vi "Robot Systems.vi"(11 "Robot Controls":T1) -> ()   [LabVIEW 2014]
uses:
  Robot Commands.ctl
panel:
  # "Field Centric"
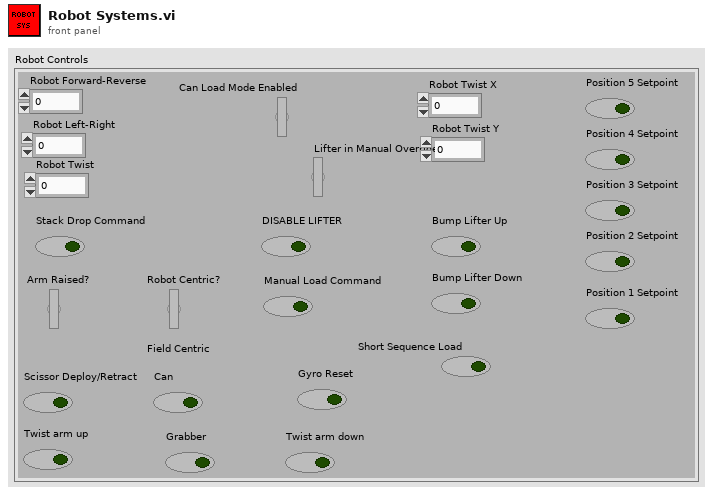
[diagram p1: front panel]
types:
  T1 = typedef "Robot Commands.ctl" = cluster{"Robot Forward-Reverse":dbl, "Robot Left-Right":dbl, "Robot Twist":dbl, "Can Load Mode Enabled":bool, "Lifter in Manual Override?":bool, "Stack Drop Command":bool, "Arm Raised?":bool, "DISABLE LIFTER":bool, "Position 1 Setpoint":bool, "Position 2 Setpoint":bool, "Position 3 Setpoint":bool, "Position 4 Setpoint":bool, "Position 5 Setpoint":bool, "Bump Lifter Down":bool, "Bump Lifter Up":bool, "Manual Load Command":bool, "Robot Centric?":bool, "Scissor Deploy/Retract":bool, "Grabber":bool, "Can":bool, "Twist arm up":bool, "Gyro Reset":bool, "Twist arm down":bool, "Short Sequence Load":bool, "Robot Twist X":dbl, "Robot Twist Y":dbl}
  T2 = typedef "Step Deployment SS State.ctl" = enum16{"Manual Override", "Disabled"}
  T3 = typedef "Stacking SS State.ctl" = enum16{"Manual Load", "Manual Override"}
  T4 = typedef "Drive SS State.ctl" = enum16{"Swerve Drive", "Arcade Drive", "Mecanum Drive"}
  T5 = typedef "Stacking SS Actuators.ctl" = cluster{"Can Solenoid":T6, "Lifter Motor":dbl, "Grabber Solenoid":T6}
  T6 = typedef "WPI_SolenoidValue.ctl" = enum16{"Off", "On", "Forward", "Reverse"}
  T7 = typedef "Drive SS Actuator Values.ctl" = cluster{"Front Left Drive Motor":dbl, "Front Left Spin Motor":dbl, "Front Right Drive Motor":dbl, "Front Right Spin Motor":dbl, "Rear Left Drive Motor":dbl, "Rear Left Spin Motor":dbl, "Rear Right Drive Motor":dbl, "Rear Right Spin Motor":dbl}
  T8 = typedef "Step Deployment Actuator Values.ctl" = cluster{"Scissors":T6}
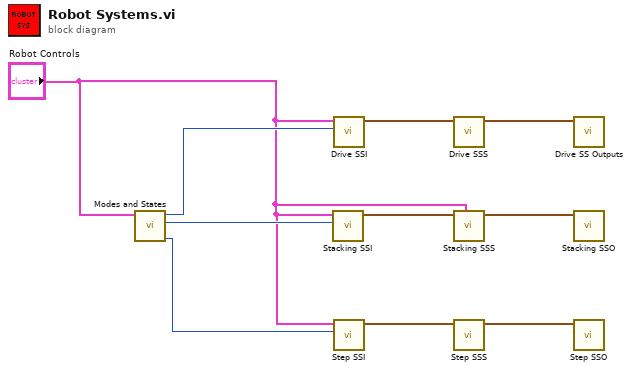
[diagram p0: block diagram]
diagram:
  n1 = call "Modes and States.vi"("Robot Controls"="Robot Controls") -> ("Step Deployment SS State"=w2:T2, "Stacking SS State"=w3:T3, "Drive SS State"=w10:T4)  [unwired: 7 in, 1 out]
  n2 = call "Stacking SSI.vi"("Stacking SS State"=w3, "Robot Controls"="Robot Controls") -> ("Stacking Actuators Out"=w4:T5)  [unwired: 9 in]
  n3 = call "Drive SSI.vi"("Drive SS State"=w10, "Robot Controls"="Robot Controls") -> ("Drive SS Actuator Values Out"=w6:T7)  [unwired: 9 in]
  n4 = call "Step SSI.vi"("Step Deployment State"=w2, "Robot Controls"="Robot Controls") -> ("Step Actuator Values Out"=w8:T8)  [unwired: 9 in]
  n5 = call "Drive SSS.vi"("Drive SS Actuator Values In"=w6) -> ("Drive SS Actuator Values Out"=w5:T7)  [unwired: 10 in]
  n6 = call "Stacking SSS.vi"("Robot Controls"="Robot Controls", "Actuator Values in"=w4) -> ("Actuator Values Out"=w9:T5)  [unwired: 9 in]
  n7 = call "Step SSS.vi"("Step Actuator Values In"=w8) -> ("Step Actuator Values Out"=w7:T8)  [unwired: 10 in]
  n8 = call "Drive SS Outputs.vi"("Drive SS Actuator Values In"=w5) -> ()  [unwired: 11 in]
  n9 = call "Stacking SSO.vi"("Actuator Values In"=w9) -> ()  [unwired: 11 in]
  n10 = call "Step SSO.vi"("Step Actuator Values In"=w7) -> ()  [unwired: 11 in]
